vi "Untitled 3.vi"() -> ()   [LabVIEW 2020]
uses:
  <vilib>/Viviota/shared/ORM_DBConnections.lvlibp/PostgresqlConnection/PostgresqlConnection.lvclass
  C:/Program Files/National Instruments/LabVIEW 2020/vi.lib/Viviota/shared/ORM.lvlibp/ORM/DbConnection/DbConnection.lvclass
  <vilib>/Viviota/shared/ORM_ADONet.lvlibp/ADOMapper/ADOMapper.lvclass
  C:/Program Files/National Instruments/LabVIEW 2020/vi.lib/Viviota/shared/ORM.lvlibp/ORM/SqlMapper/SqlMapper.lvclass
  <vilib>/Viviota/shared/ORM.lvlibp/ORM/TypeMap/TypeMap.lvclass
  de15e16b-8ab6-4424-bedc-11d304f59ddd.vi
  20b45f6d-0a41-487a-a6b2-240acaf8d124.vi
  <vilib>/Utility/High Resolution Relative Seconds.vi
  de15e16b-8ab6-4424-bedc-11d304f59ddd.vi/35b31214-e0d6-4ae0-b34c-13eba9df70db.vi
  de15e16b-8ab6-4424-bedc-11d304f59ddd.vi/2e8f1eab-5a58-47e6-9224-d0a2895e31fd.vi
  20b45f6d-0a41-487a-a6b2-240acaf8d124.vi/35b31214-e0d6-4ae0-b34c-13eba9df70db.vi
  20b45f6d-0a41-487a-a6b2-240acaf8d124.vi/2e8f1eab-5a58-47e6-9224-d0a2895e31fd.vi
  <userlib>/_OpenG.lib/file/file.llb/Convert File Extension (Path)__ogtk.vi
  <vilib>/Viviota/shared/ORM.lvlibp/ORM/SqlMapper/Write DbConnection.vi
  <vilib>/Utility/error.llb/Error Cluster From Error Code.vi
  <vilib>/Viviota/shared/ORM.lvlibp/ORM/TypeMap/Write Table Name.vi
  <vilib>/Viviota/shared/ORM.lvlibp/ORM/TypeMap/Write Autokey.vi
  <vilib>/Viviota/shared/ORM.lvlibp/ORM/SqlMapper/End Transaction.vi
  <vilib>/Viviota/shared/ORM.lvlibp/ORM/SqlMapper/SqlMapper.lvclass
  <vilib>/Viviota/VIV_Tools/Helpers.lvlib
  <vilib>/Viviota/shared/ORM_lib.lvlibp/ObjectRow/ObjectLUT.lvclass
panel:
  out "Difference 3":dbl
  out "Difference 2":dbl
  out "Difference":dbl
  out "id 2":i32
  out "id":i32
  out "Variant":variant
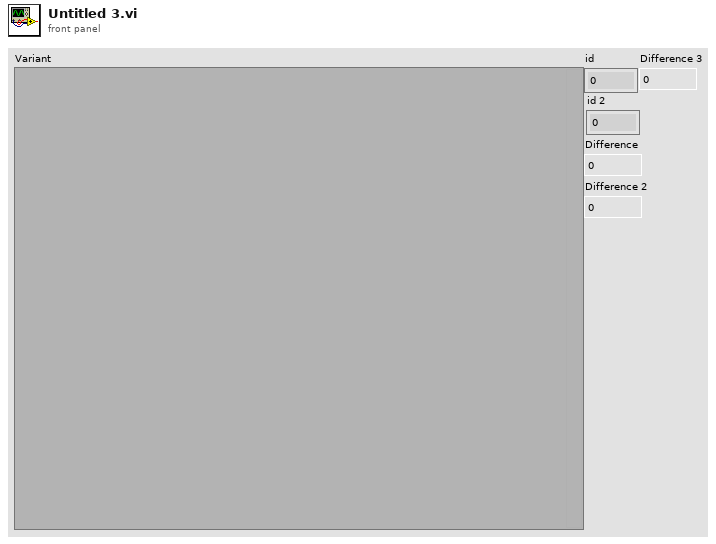
[diagram p1: front panel]
types:
  T1 = enum16{"open", "open or create", "create or replace", "create", "open (read-only)"}
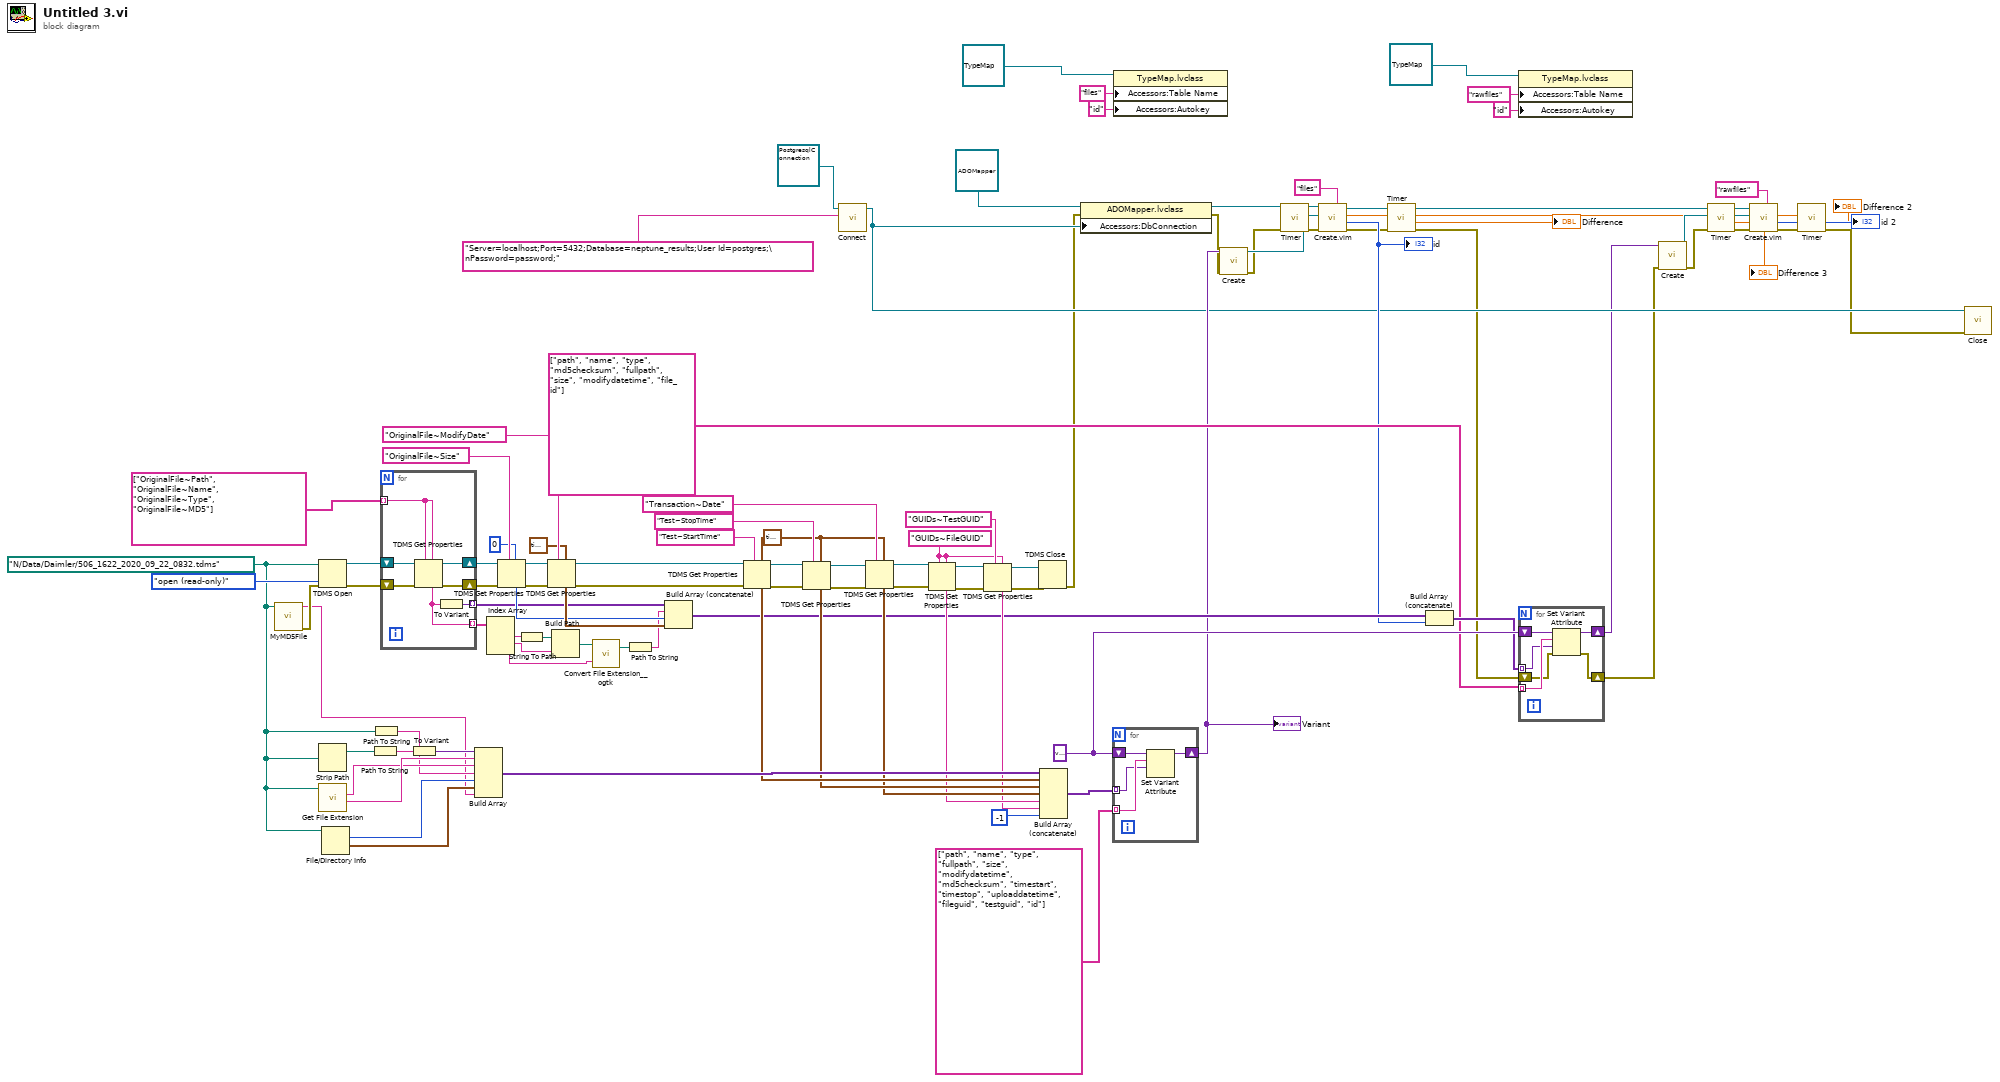
[diagram p0: block diagram]
diagram:
  w42 = variant ("Variant")
  w63 = "GUIDs~FileGUID" ("property name")
  w65 = timestamp(0 s since 1904-01-01) ("Timestamp")
  w71 = path "N:/Data/Daimler/506_1622_2020_09_22_0832.tdms"
  n1 = call <vilib>:"MyMD5File.vi"("File"=w71) -> ("error out"=w70:errorcluster, "MD5"=w69:string)  [unwired: 9 in]
  n2 = TDMS Open(8:w70, 10:T1."open (read-only)" ("operation (0:open)"), 11:w71) -> (0:w100:errorcluster, 3:w101:refnum<k34>)  [unwired: 4 in]
  n3 = Strip Path(path=w71) -> (stripped path=w79:path)  [unwired: 1 out]
  n4 = call <vilib>:"Get File Extension.vi"("file"=w71) -> ("filename without extension"=w77:string, "lowercase file extension"=w76:string)  [unwired: 6 in, 3 out]
  n5 = File/Directory Info(path=w71) -> (size=w73:i64, last mod=w72:timestamp)  [unwired: 1 in, 5 out]
  n6 = Path To String(path=w79) -> (string=w78:string)
  n7 = Path To String(path=w71) -> (string=w75:string)
  n8 = for {
    tunnel: string[] ["OriginalFile~Path", "OriginalFile~Name", "OriginalFile~Type", "OriginalFile~MD5"] -> [w107] mode=indexing
    tunnel: [w104] -> w84 mode=indexing
    shift-right: [w106] -> w98
    shift-left: w101 -> [w109]
    shift-right: [w105] -> w97
    shift-left: w100 -> [w108]
    tunnel: [w103] -> w88 mode=indexing
    n9 = TDMS Get Properties(5:w107, 7:w107, 8:w108, 11:w109) -> (0:w105:errorcluster, 3:w106:refnum<k34>, 4:w103:string)  [unwired: 2 in, 3 out]
    n10 = To Variant(anything=w103) -> (Variant=w104:variant)
  }
  n11 = To Variant(anything=w78) -> (Variant=w74:variant)
  n12 = Build Array(w74, w77, w76, w75, w73, w72, w69) -> (w62:variant[])
  n13 = Index Array(array=w88) -> (element #1=w87:string, element #2=w85:string, element #3=w82:string)  [unwired: 3 in]
  n14 = TDMS Get Properties(5:i64 0, 7:"OriginalFile~Size", 8:w97, 11:w98) -> (0:w92:errorcluster, 3:w91:refnum<k34>, 4:w89:i64)  [unwired: 2 in, 3 out]
  n15 = String To Path(string=w87) -> (path=w86:path)
  n16 = TDMS Get Properties(5:timestamp(0 s since 1904-01-01) ("Timestamp"), 7:"OriginalFile~ModifyDate", 8:w92, 11:w91) -> (0:w60:errorcluster, 3:w61:refnum<k34>, 4:w90:timestamp)  [unwired: 2 in, 3 out]
  n17 = Build Path(base path=w86, name or relative path=w85) -> (appended path=w83:path)
  n18 = call-poly <userlib>:"Convert File Extension__ogtk.vi"("new ending (none)"=w82, "file name"=w83) -> ("new filename"=w81:path)  [unwired: 1 out]
  n19 = Path To String(path=w81) -> (string=w80:string)
  n20 = Build Array (concatenate)(w84, w80, w89, w90) -> (w41:variant[])
  n21 = TDMS Get Properties(5:w65, 7:"Test~StartTime" ("property name"), 8:w60, 11:w61) -> (0:w58:errorcluster, 3:w59:refnum<k34>, 4:w49:timestamp)  [unwired: 2 in, 3 out]
  n22 = TDMS Get Properties(5:w65, 7:"Test~StopTime" ("property name"), 8:w58, 11:w59) -> (0:w56:errorcluster, 3:w57:refnum<k34>, 4:w48:timestamp)  [unwired: 2 in, 3 out]
  n23 = call-dynamic "Connect.vi"("Connection String"="Server=localhost;Port=5432;Database=neptune_results;User Id=postgres;\nPassword=password;", "PostgresqlConnection in"=refnum<class "PostgresqlConnection.lvclass"> refnum) -> ("PostgresqlConnection out"=w28:refnum<class "PostgresqlConnection.lvclass">)  [unwired: 8 in, 1 out]
  n24 = TDMS Get Properties(5:w65, 7:"Transaction~Date" ("property name"), 8:w56, 11:w57) -> (0:w54:errorcluster, 3:w55:refnum<k34>, 4:w47:timestamp)  [unwired: 2 in, 3 out]
  n25 = TDMS Get Properties(5:w63, 7:w63, 8:w54, 11:w55) -> (0:w52:errorcluster, 3:w53:refnum<k34>, 4:w46:string)  [unwired: 2 in, 3 out]
  n26 = TDMS Get Properties(5:w63, 7:"GUIDs~TestGUID" ("property name"), 8:w52, 11:w53) -> (0:w50:errorcluster, 3:w51:refnum<k34>, 4:w45:string)  [unwired: 2 in, 3 out]
  n27 = TDMS Close(8:w50, 11:w51) -> (0:w15:errorcluster)  [unwired: 1 out]
  n28 = Build Array (concatenate)(w62, w49, w48, w47, w46, w45, -1) -> (w44:variant[])
  n29 = property class="ADOMapper.lvclass"(reference=refnum<class "ADOMapper.lvclass"> refnum ("ADONet.lvlib:ADOMapper.lvclass"), error in=w15, "Accessors:DbConnection"=w28) -> (reference out=w32:refnum<class "ADOMapper.lvclass">, error out=w12:errorcluster)
  n30 = for {
    tunnel: w44 -> [w110] mode=indexing
    shift-right: [w112] -> w35
    shift-left: w42 -> [w113]
    tunnel: string[] ["path", "name", "type", "fullpath", "size", "modifydatetime", "md5checksum", "timestart", "timestop", "uploaddatetime", "fileguid", "testguid", "id"] -> [w111] mode=indexing
    n31 = Set Variant Attribute(Variant=w113, name=w111, value=w110) -> (Variant out=w112:variant)  [unwired: 1 in, 2 out]
  }
  "Variant" <- w35
  n32 = property class="TypeMap.lvclass"(reference=refnum<class "TypeMap.lvclass"> refnum ("ORM.lvlibp:TypeMap.lvclass"), "Accessors:Table Name"="files" ("Table Name"), "Accessors:Autokey"="id" ("Autokey")) -> ()  [unwired: 1 in, 2 out]
  n33 = call <vilib>:"Create.vi"("error in"=w12, "LUT"=w35) -> ("error out"=w11:errorcluster, "ORM_lib.lvlib:ObjectLUT.lvclass"=w34:refnum<class "ObjectLUT.lvclass">)  [unwired: 8 in]
  n34 = call <vilib>:"Timer.vi"("error in (no error)"=w11) -> ("error out"=w20:errorcluster, "Current Time"=w18:dbl)  [unwired: 4 in, 1 out]
  n35 = call "Create.vim"("TypeMap in"="files", "error in (no error)"=w20, "object in"=w34, "SqlMapper in"=w32) -> ("error out"=w10:errorcluster, "id"=w29:i32, "SqlMapper out"=w27:refnum<class "SqlMapper.lvclass">)  [unwired: 4 in, 1 out]
  "id" <- w29
  n36 = call <vilib>:"Timer.vi"("error in (no error)"=w10, "Last Time"=w18) -> ("error out"=w8:errorcluster, "Difference"=→"Difference":dbl, "Current Time"=w4:dbl)  [unwired: 3 in]
  n37 = Build Array (concatenate)(w41, w29) -> (w40:variant[])
  n38 = property class="TypeMap.lvclass"(reference=refnum<class "TypeMap.lvclass"> refnum ("ORM.lvlibp:TypeMap.lvclass"), "Accessors:Table Name"="rawfiles" ("Table Name"), "Accessors:Autokey"="id" ("Autokey")) -> ()  [unwired: 1 in, 2 out]
  n39 = for {
    tunnel: w40 -> [w116] mode=indexing
    shift-right: [w118] -> w24
    shift-left: w42 -> [w119]
    tunnel: string[] ["path", "name", "type", "md5checksum", "fullpath", "size", "modifydatetime", "file_id"] -> [w117] mode=indexing
    shift-right: [w114] -> w9
    shift-left: w8 -> [w115]
    n40 = Set Variant Attribute(Variant=w119, name=w117, value=w116, error in=w115) -> (Variant out=w118:variant, error out=w114:errorcluster)  [unwired: 1 out]
  }
  n41 = call <vilib>:"Create.vi"("error in"=w9, "LUT"=w24) -> ("error out"=w7:errorcluster, "ORM_lib.lvlib:ObjectLUT.lvclass"=w23:refnum<class "ObjectLUT.lvclass">)  [unwired: 8 in]
  n42 = call <vilib>:"Timer.vi"("error in (no error)"=w7, "Last Time"=w4) -> ("error out"=w6:errorcluster, "Difference"=→"Difference 3":dbl, "Current Time"=w5:dbl)  [unwired: 3 in]
  n43 = call "Create.vim"("TypeMap in"="rawfiles", "error in (no error)"=w6, "object in"=w23, "SqlMapper in"=w27) -> ("error out"=w21:errorcluster, "id"=→"id 2":i32)  [unwired: 4 in, 2 out]
  n44 = call <vilib>:"Timer.vi"("error in (no error)"=w21, "Last Time"=w5) -> ("error out"=w19:errorcluster, "Difference"=→"Difference 2":dbl)  [unwired: 3 in, 1 out]
  n45 = call-dynamic "Close.vi"("error in (no error)"=w19, "DbConnection in"=w28) -> ()  [unwired: 9 in, 1 out]
